vi "Display.vi"(11 "Display Data":refnum<class "Display Data.lvclass">) -> ()   [LabVIEW 2013, in "Display Data.lvclass"]
uses:
  Display Data.lvclass
  Display Data.lvclass/Display Data.ctl
  State data/State Data.lvclass/State Data.ctl
  State data/Read Extinction.vi
  State data/Read IA.vi
  <vilib>/Analysis/6fits.llb/Prediction Interval (Linear).vi
  <vilib>/Analysis/NI_AALPro.lvlib
  State data/State Data.lvclass
panel:
  out "r2":dbl
  out "b":dbl
  out "m":dbl
  in  "Accept Cal":bool
  out "seconds":u8 caption="Seconds Until Accept"
  out "Calibration Plot":cluster{dbl[], "Best Linear Fit":dbl[]}[](graph)
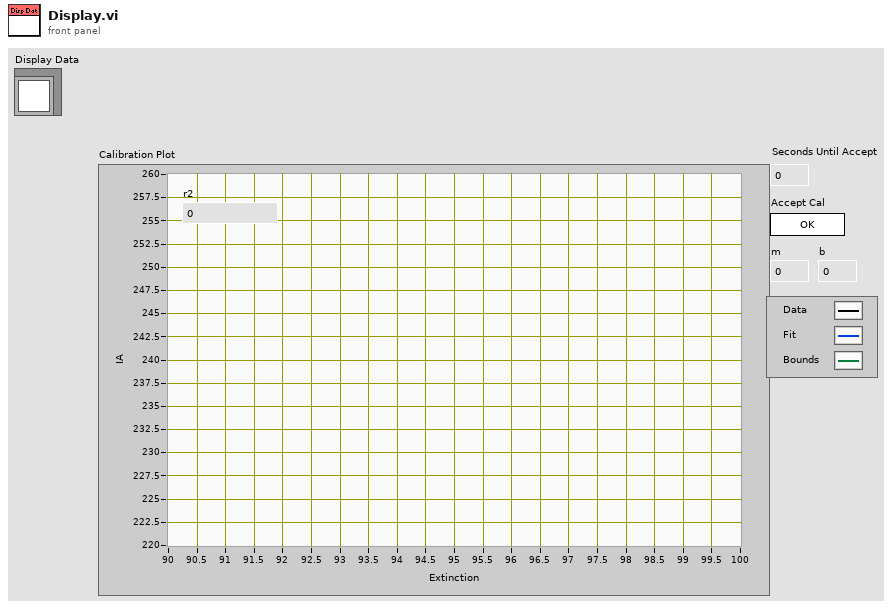
[diagram p1: front panel]
types:
  T1 = cluster{"Stored State":refnum<class "State Data.lvclass">[], "pointer to data":i32}
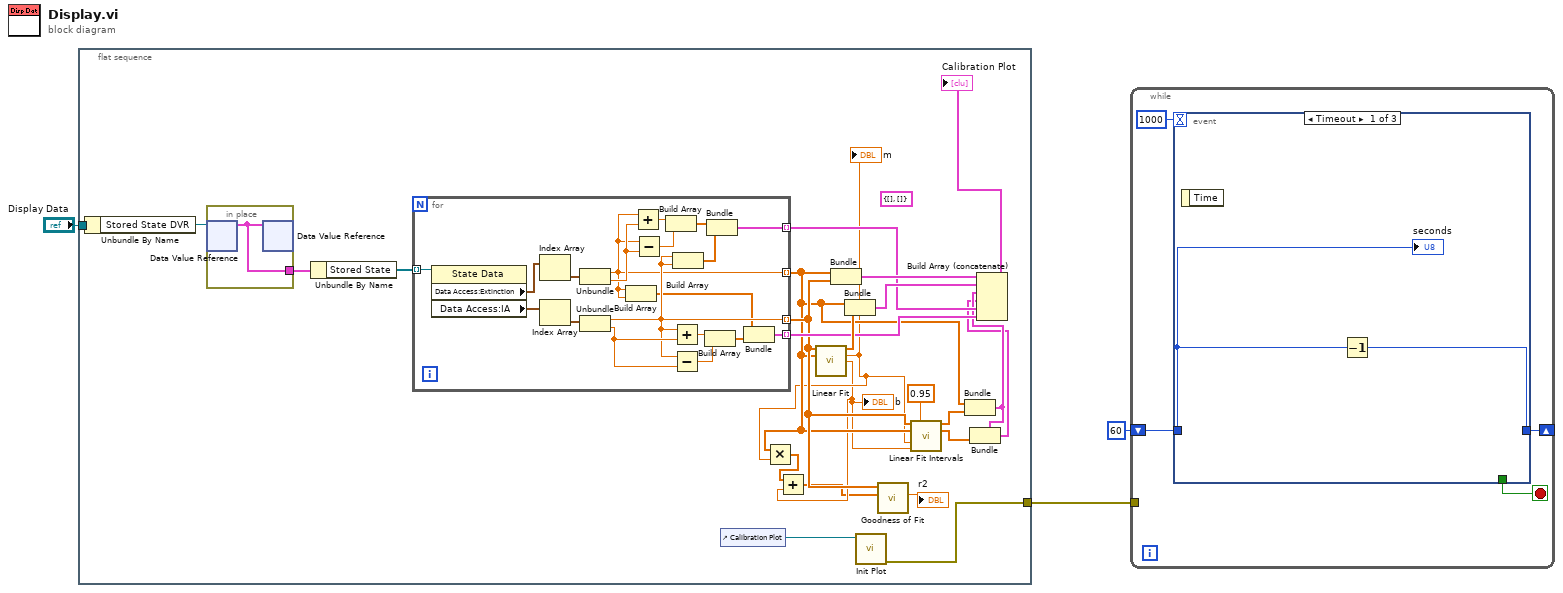
[diagram p0: block diagram]
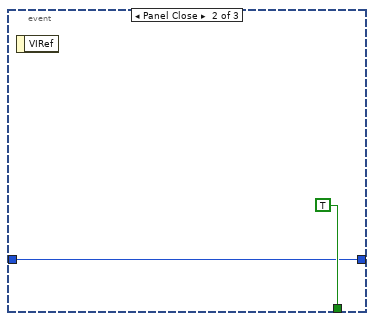
[diagram p2: hidden frame]
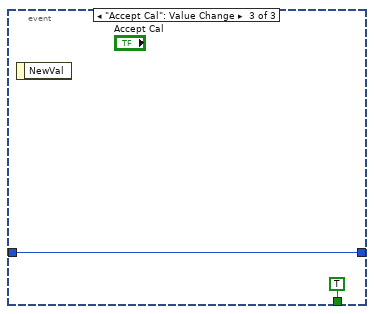
[diagram p3: hidden frame]
diagram:
  n1 = flat-sequence {
    tunnel: "Display Data" -> [w27]
    tunnel: [w18] -> w1
    frame #0 {
      (unwired) cluster{dbl[], "Best Linear Fit":dbl[]} {[], "Best Linear Fit"=[]} ("element")
      n2 = Unbundle By Name(w27) -> ("Stored State DVR"=w26:refnum<data-value>)
      n3 = in-place {
        in-place-border: [w47] -> w17
        n4 = in-place-dvr #1(w26) -> (w47:T1)  [unwired: 1 out]
        n5 = in-place-dvr #1(w47) -> ()  [unwired: 2 out]
      }
      n6 = Unbundle By Name(w17) -> ("Stored State"=w16:refnum<class "State Data.lvclass">[])
      n7 = for {
        tunnel: w16 -> [w46] mode=indexing
        tunnel: [w37] -> w9 mode=indexing
        tunnel: [w41] -> w10 mode=indexing
        tunnel: [w38] -> w22 mode=indexing
        tunnel: [w32] -> w21 mode=indexing
        n8 = property class="State Data"(reference=w46) -> ("Data Access:Extinction"=w31:cluster{"Mean":dbl, "Error":dbl}[], "Data Access:IA"=w29:cluster{"Mean":dbl, "Error":dbl}[])  [unwired: 1 in, 2 out]
        n9 = Index Array(array=w31) -> (element=w30:cluster{"Mean":dbl, "Error":dbl})  [unwired: 1 in]
        n10 = Index Array(array=w29) -> (element=w28:cluster{"Mean":dbl, "Error":dbl})  [unwired: 1 in]
        n11 = Unbundle(w30) -> ("Mean"=w37:dbl, "Error"=w45:dbl)
        n12 = Unbundle(w28) -> ("Mean"=w41:dbl, "Error"=w44:dbl)
        n13 = Build Array(w37, w37) -> (w34:dbl[])
        n14 = Add(x=w37, y=w45) -> (x+y=w42:dbl)
        n15 = Subtract(x=w37, y=w45) -> (x-y=w43:dbl)
        n16 = Build Array(w42, w43) -> (w39:dbl[])
        n17 = Add(x=w41, y=w44) -> (x+y=w36:dbl)
        n18 = Subtract(x=w41, y=w44) -> (x-y=w35:dbl)
        n19 = Build Array(w41, w41) -> (w40:dbl[])
        n20 = Build Array(w36, w35) -> (w33:dbl[])
        n21 = Bundle(w39, w40) -> (w38:cluster{dbl[], dbl[]})  [unwired: 1 in]
        n22 = Bundle(w34, w33) -> (w32:cluster{dbl[], dbl[]})  [unwired: 1 in]
      }
      n23 = control-ref of="Calibration Plot"() -> (w20:refnum<vi>)
      n24 = call <vilib>:"Linear Fit.vi"("Y"=w10, "X"=w9) -> ("Best Linear Fit"=w25:dbl[], "slope"=w8:dbl, "intercept"=w6:dbl)  [unwired: 9 in, 2 out]
      "m" <- w8
      "b" <- w6
      n25 = Multiply(x=w9, y=w8) -> (x*y=w7:dbl[])
      n26 = Add(x=w7, y=w6) -> (x+y=w5:dbl[])
      n27 = Bundle(w9, w10) -> (w24:cluster{dbl[], dbl[]})  [unwired: 1 in]
      n28 = Bundle(w9, "Best Linear Fit"=w25) -> (w23:cluster{dbl[], "Best Linear Fit":dbl[]})  [unwired: 1 in]
      n29 = call "Init Plot.vi"("XYGraph in"=w20) -> ("error out"=w18:errorcluster)  [unwired: 10 in]
      n30 = call <vilib>:"Goodness of Fit.vi"("Best Fit"=w5, "Y"=w10) -> ("R-square"=→"r2":dbl)  [unwired: 6 in, 3 out]
      n31 = call-poly <vilib>:"Linear Fit Intervals.vi"("Y"=w10, "confidence level"=0.95, "X"=w9, "slope"=w8, "intercept"=w6) -> ("Upper Bound"=w14:dbl[], "Lower Bound"=w13:dbl[])  [unwired: 8 in, 1 out]
      n32 = Bundle(w9, "Upper Bound"=w14) -> (w12:cluster{dbl[], "Upper Bound":dbl[]})  [unwired: 1 in]
      n33 = Bundle(cluster=w12, "Upper Bound"=w13) -> (w11:cluster{dbl[], "Upper Bound":dbl[]})  [unwired: 1 in]
      n34 = Build Array (concatenate)(w24, w23, w12, w11, w22, w21) -> (→"Calibration Plot":cluster{dbl[], "Upper Bound":dbl[]}[])
    }
  }
  n35 = while {
    shift-right: [w48] -> _
    shift-left: u8 60 -> [w49]
    tunnel: w1 -> [_]
    stop <- w51 stop-if-true
    n36 = event shown="[0] Timeout" {
      selector: _ -> [_ _ _]
      dyn-events: _ -> [_ _ _]
      timeout: 1000 -> [_ _ _]
      tunnel: [_ TRUE TRUE] -> w51
      tunnel: w49 -> [w53 w54 w56]
      tunnel: [w52 w54 w56] -> w48
      event Timeout {
        n37 = event-data() -> ()  [unwired: 1 in, 1 out]
        n38 = Decrement(x=w53) -> (x-1=w52:u8)
        "seconds" <- w53
      }
      event Panel Close {
        n39 = event-data() -> ()  [unwired: 1 in, 1 out]
      }
      event "Accept Cal": Value Change {
        n40 = event-data() -> ()  [unwired: 1 in, 1 out]
      }
    }
  }
